vi "Func_AddToEnum.vi"(8 "error in (no error)":errorcluster, 10 "data type name":string, 11 "VI in":refnum<vi>) -> (0 "error out":errorcluster, 3 "NumItems":u32)   [LabVIEW 2010, in "TemplateGenerator.lvlib"]
uses:
  TemplateGenerator.lvlib
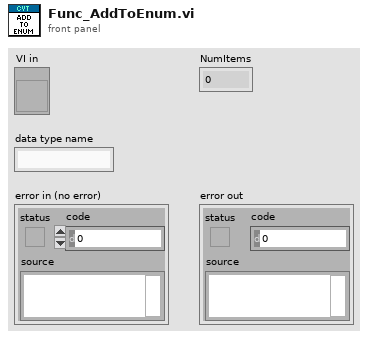
[diagram p1: front panel]
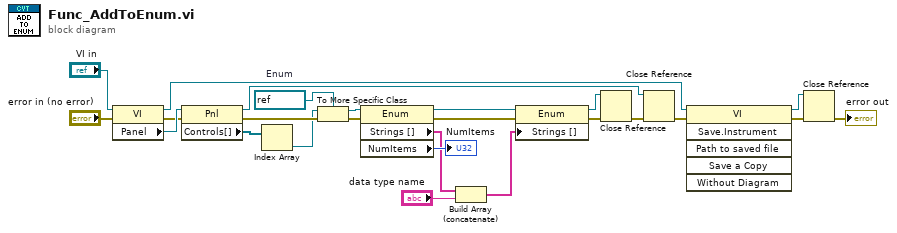
[diagram p0: block diagram]
diagram:
  w9 = refnum<vi> refnum  # Enum
  n1 = property class="VI"(reference="VI in", error in="error in (no error)") -> (reference out=w1:refnum<vi>, error out=w10:errorcluster, "Panel"=w14:refnum<vi>)
  n2 = property class="Pnl"(reference=w14, error in=w10) -> (reference out=w11:refnum<vi>, error out=w13:errorcluster, "Controls[]"=w6:refnum<vi>[])
  n3 = Index Array(array=w6) -> (element=w5:refnum<vi>)  [unwired: 1 in]
  n4 = To More Specific Class(target class=w9, reference=w5, error in=w13) -> (specific class reference=w8:refnum<vi>, error out=w7:errorcluster)
  n5 = property class="Enum"(reference=w8, error in=w7) -> (reference out=w16:refnum<vi>, error out=w19:errorcluster, "Strings []"=w20:string[], "NumItems"=→"NumItems":u32)
  n6 = Build Array (concatenate)(w20, "data type name") -> (w21:string[])
  n7 = property class="Enum"(reference=w16, error in=w19, "Strings []"=w21) -> (reference out=w17:refnum<vi>, error out=w18:errorcluster)
  n8 = Close Reference(reference=w17, error in (no error)=w18) -> (error out=w12:errorcluster)
  n9 = Close Reference(reference=w11, error in (no error)=w12) -> (error out=w4:errorcluster)
  n10 = invoke class="VI" method="Save.Instrument"(reference=w1, error in=w4) -> (reference out=w2:refnum<vi>, error out=w3:errorcluster)  [unwired: 4 in, 4 out]
  n11 = Close Reference(reference=w2, error in (no error)=w3) -> (error out=→"error out":errorcluster)
